vi "Create Trigger.vi"(11 "error in (no error)":errorcluster) -> (4 "Queue out":refnum<queue>, 15 "error out":errorcluster)   [LabVIEW 2015, in "TLB` Template.lvlib"]
uses:
  TLB` Template.lvlib
  System Trigger Element.ctl
  System Trigger.ctl
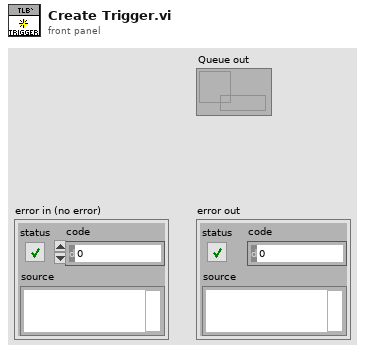
[diagram p1: front panel]
types:
  T1 = typedef "TLB` Template.lvlib/System Trigger Element.ctl" = cluster{"System Triggers":T2, "Trigger Data":variant}
  T2 = typedef "TLB` Template.lvlib/System Trigger.ctl" = enum16{"<None>", "Cache User Parameters", "Close Application"}
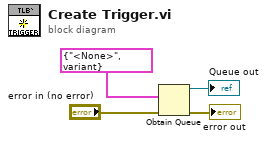
[diagram p0: block diagram]
diagram:
  n1 = Obtain Queue(element data type=T1 {"System Triggers"=enum."<None>", "Trigger Data"=variant} ("element"), error in (no error)="error in (no error)") -> (queue out=→"Queue out":refnum<queue>, error out=→"error out":errorcluster)  [unwired: 3 in, 1 out]
